vi "DataRecord_SubVi.vi"(0 "string":string, 1 "Array":dbl[](array[numeric]), 2 "File Path":string="D:\\Dropbox\\MResMedicalRobotics\\MResIndivisualProject\\Arduino\\Labview\\CTR Project\\data\\") -> ()   [LabVIEW 2015]
uses:
  <vilib>/Utility/file.llb/Write To Spreadsheet File (DBL).vi
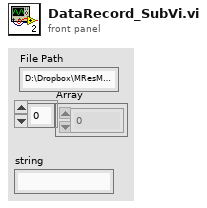
[diagram p1: front panel]
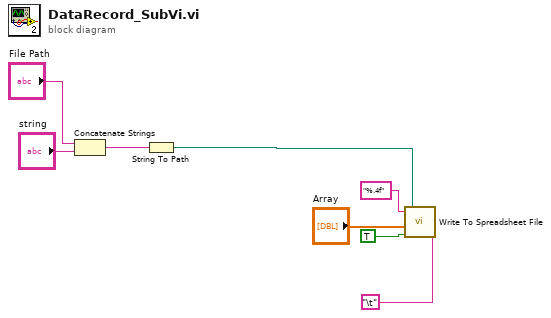
[diagram p0: block diagram]
diagram:
  n1 = Concatenate Strings("File Path", "string") -> (w6:string)
  n2 = String To Path(string=w6) -> (path=w2:path)
  n3 = call-poly <vilib>:"Write To Spreadsheet File.vi"("delimiter (\\t)"="\t", "format (%.3f)"="%.4f", "append to file? (new file:F)"=TRUE, "1D data"="Array", "file path (dialog if empty)"=w2) -> ()  [unwired: 3 in, 1 out]
